vi "Write Voltage Scale.vi"(8 "error in (no error)":errorcluster, 10 "Voltage Scale":dbl, 11 "BigMAQ in":refnum<class "BigMAQ.lvclass">) -> (0 "error out":errorcluster, 3 "BigMAQ out":refnum<class "BigMAQ.lvclass">)   [LabVIEW 2019, in "BigMAQ.lvclass"]
uses:
  BigMAQ.lvclass
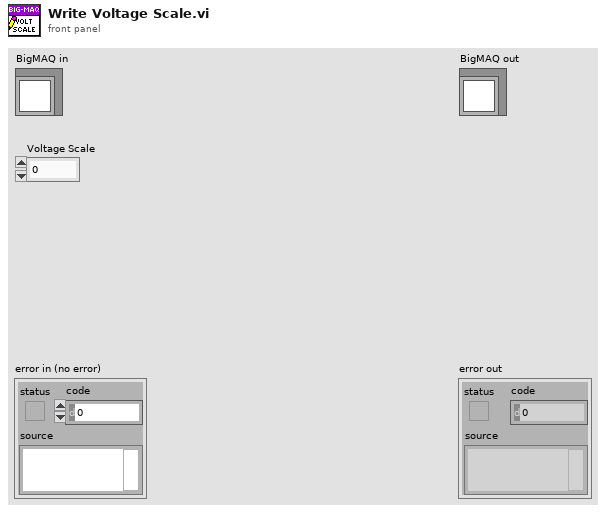
[diagram p1: front panel]
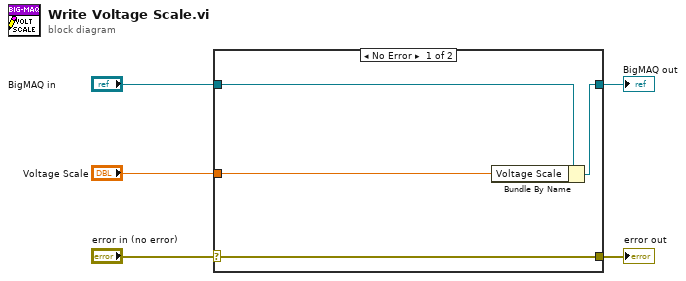
[diagram p0: block diagram]
diagram:
  n1 = case shown="No Error" "error in (no error)" {
    selector: "error in (no error)" -> [w9 w10]
    tunnel: [w9 w10] -> w4
    tunnel: [w7 w11] -> w2
    tunnel: "BigMAQ in" -> [w8 w11]
    tunnel: "Voltage Scale" -> [w6 _]
    frame No Error {
      n2 = Bundle By Name(cluster=w8, "Voltage Scale"=w6) -> (w7:refnum<class "BigMAQ.lvclass">)
    }
    frame Error {
    }
  }
  "error out" <- w4
  "BigMAQ out" <- w2
